vi "Create from Folder (Factory).vi"(8 "error in (no error)":errorcluster, 9 "Name (type:folder)":string, 10 "Folder":path) -> (0 "error out":errorcluster, 3 "PackageAbstract out":refnum<class "PackageAbstract.lvclass">)   [LabVIEW 2020, in "GPack.lvlib" / "PackageAbstract.lvclass"]
uses:
  PackageAbstract.lvclass
  C:/dev/lv20CE/lv-gpack/GPack/Package/Package.lvclass
  GPack File/GPack File.lvclass
  PackageAbstract.lvclass/PackageAbstract.ctl
  GPack.lvlib
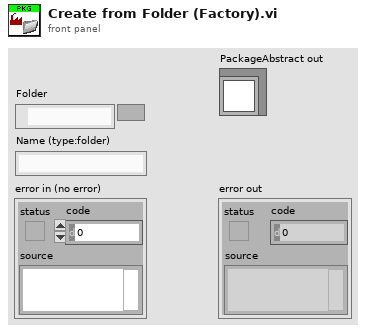
[diagram p1: front panel]
types:
  T1 = typedef "GPack.lvlib/Package Info.ctl" = cluster{"Name":string, "Type":string, "Source":string, "Branch":string, "Version":string}
  T2 = typedef "GPack.lvlib/Dependency.ctl" = cluster{"Info":T1, "Path":path}
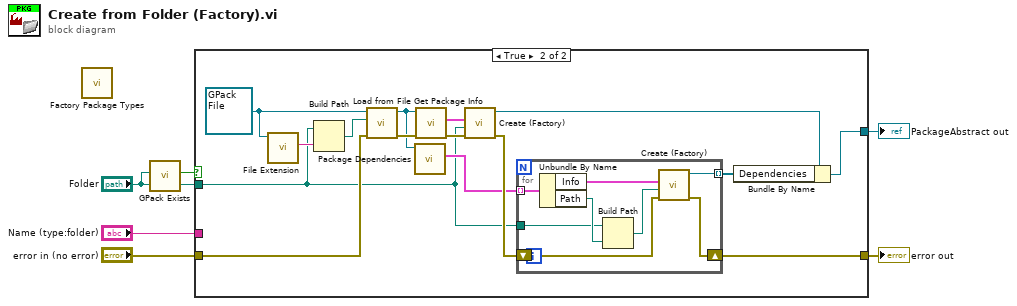
[diagram p0: block diagram]
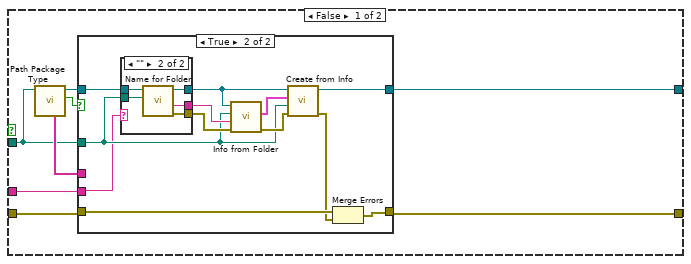
[diagram p2: hidden frame]
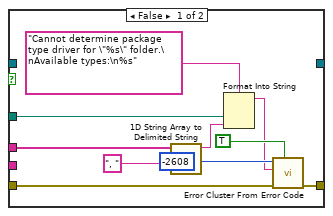
[diagram p3: hidden frame]
diagram:
  n1 = call "Factory Package Types.vi"() -> ()  [unwired: 12 in]
  n2 = call "GPack Exists.vi"("Folder"="Folder") -> ("Has GPack"=w1:bool)  [unwired: 10 in]
  n3 = case shown="True" w1 {
    tunnel: "error in (no error)" -> [w14 w52]
    tunnel: [w13 w45] -> w5
    tunnel: [w12 w46] -> w4
    tunnel: "Name (type:folder)" -> [w8 _]
    tunnel: "Folder" -> [w7 w44]
    frame False {
      n4 = call "Path Package Type.vi"("Path"=w7) -> ("Matched"=w9:bool, "First Match"=w10:refnum<class "PackageAbstract.lvclass">, "Available Types"=w11:string[])  [unwired: 7 in, 1 out]
      n5 = case shown="True" w9 {
        tunnel: w14 -> [w24 w29]
        tunnel: w10 -> [_ w36]
        tunnel: w7 -> [w20 w26]
        tunnel: [w22 w27] -> w13
        tunnel: [_ w30] -> w12
        tunnel: w11 -> [w15 _]
        tunnel: w8 -> [_ w25]
        frame False {
          n6 = call <vilib>:"1D String Array to Delimited String.vi"("delimiter"=", ", "string array"=w15) -> ("delimited string"=w18:string)  [unwired: 9 in]
          n7 = Format Into String(format string="Cannot determine package type driver for \"%s\" folder.\nAvailable types:\n%s", w20, w18) -> (resulting string=w16:string)  [unwired: 2 in, 1 out]
          n8 = call <vilib>:"Error Cluster From Error Code.vi"("show call chain? (False)"=TRUE, "error in (no error)"=w24, "error message (\"\")"=w16, "error code (0)"=-2608) -> ("error out"=w22:errorcluster)  [unwired: 5 in]
        }
        frame True {
          n9 = case shown="\"\"" w25 {
            selector: w25 -> [w37 _]
            tunnel: w36 -> [w38 w43]
            tunnel: [w37 w42] -> w35
            tunnel: [_ w41] -> w34
            tunnel: [w38 w40] -> w31
            tunnel: w26 -> [_ w39]
            frame Default {
            }
            frame "" {
              n10 = call "Name for Folder.vi"("Folder"=w39, "PackageAbstract in"=w43) -> ("error out"=w41:errorcluster, "Name"=w42:string, "PackageAbstract out"=w40:refnum<class "PackageAbstract.lvclass">)  [unwired: 6 in, 1 out]
            }
          }
          n11 = call-dynamic "Info from Folder.vi"("error in (no error)"=w34, "Name"=w35, "Folder"=w26, "Package in"=w31) -> ("error out"=w33:errorcluster, "Package Info"=w32:T1)  [unwired: 6 in]
          n12 = call-dynamic "Create from Info.vi"("error in (no error)"=w33, "Folder"=w26, "Package Info"=w32, "Package in"=w31) -> ("error out"=w28:errorcluster, "Package out"=w30:refnum<class "PackageAbstract.lvclass">)  [unwired: 6 in]
          n13 = Merge Errors(w29, w28) -> (w27:errorcluster)
        }
      }
    }
    frame True {
      w54 = refnum<class "GPack File.lvclass"> refnum ("GPack File in")
      n14 = call-dynamic "File Extension.vi"("GPack File in"=w54) -> ("File Extension"=w55:string)  [unwired: 9 in, 1 out]
      n15 = Build Path(base path=w44, name or relative path=w55) -> (appended path=w53:path)
      n16 = call-dynamic "Load from File.vi"("error in (no error)"=w52, "Path"=w53, "GPack File in"=w54) -> ("error out"=w56:errorcluster, "GPack File out"=w50:refnum<class "GPack File.lvclass">)  [unwired: 7 in]
      n17 = call-dynamic "Package Dependencies.vi"("GPack File in"=w50) -> ("Dependencies"=w49:T2[])  [unwired: 9 in, 1 out]
      n18 = call "Get Package Info.vi"("GPack File in"=w50) -> ("Package Info"=w51:T1)  [unwired: 10 in]
      n19 = call "Create (Factory).vi"("error in (no error)"=w56, "Folder"=w44, "Package Info"=w51) -> ("error out"=w57:errorcluster, "PackageAbstract out"=w48:refnum<class "PackageAbstract.lvclass">)  [unwired: 7 in]
      n20 = for {
        tunnel: w49 -> [w65] mode=indexing
        shift-right: [w62] -> w45
        shift-left: w57 -> [w63]
        tunnel: [w61] -> w47 mode=indexing
        tunnel: w44 -> [w58]
        n21 = Unbundle By Name(w65) -> ("Info"=w64:T1, "Path"=w60:path)
        n22 = Build Path(base path=w58, name or relative path=w60) -> (appended path=w59:path)
        n23 = call "Create (Factory).vi"("error in (no error)"=w63, "Folder"=w59, "Package Info"=w64) -> ("error out"=w62:errorcluster, "PackageAbstract out"=w61:refnum<class "PackageAbstract.lvclass">)  [unwired: 7 in]
      }
      n24 = Bundle By Name(cluster=w48, "Dependencies"=w47) -> (w46:refnum<class "PackageAbstract.lvclass">)
    }
  }
  "error out" <- w5
  "PackageAbstract out" <- w4
